vi "SERIAL_StartStreamCommand.vi"(11 "navX Ref":T1={"SerialPortRef"={"DevStatus"={"status"=FALSE, "code"=0, "source"=""}, "Serial Port Name"=""}, "Board Information"={"WhoAmI (50 | 0x32)"=0, "Board Revision"=0, "Firmware Major Version"=0, "Firmware Minor Version"=0, "NAVX_BOARD_CAPABILITY"={"OMNIMOUNT"=FALSE, "YAW_RESET"=FALSE, "VEL_AND_DISP"=FALSE}, "NAVX_BOARD_YAW_AXIS"={"BOARD_YAW_AXIS_UP"=FALSE, "BOARD_YAW_AXIS"=0}}, "Status"={"Update Rate Hz"=0, "Accelerometer Full-Scale Range"=0, "Gyro Full-Scale Range"=0, "NAVX_OP_STATUS"=0, "NAVX_CAL_STATUS"=0, "NAVX_SELFTEST_STATUS"=0, "NAVX_SENSOR_STATUS"={"MOVING"=FALSE, "YAW_STABLE"=FALSE, "MAG_DISTURBANCE"=FALSE, "ALTITUDE_VALID"=FALSE, "SEALEVEL_PRESS_SET"=FALSE, "FUSED_HEADING_VALID"=FALSE}}, "Offsets"={"Yaw"=0.0, "Quat W"=0.0, "Quat X"=0.0, "Quat Y"=0.0, "Quat Z"=0.0}, "Update Rate (4Hz-60Hz)"=50, "Nav6Mode (YPR)"=enum."Raw", "refnum name"="", "error"={"status"=FALSE, "code"=0, "source"=""}, "Loop VI Refnum"=refnum} {"Status"."NAVX_OP_STATUS" items=["INITIALIZING", "SELFTEST_IN_PROGRESS", "ERROR", "IMU_AUTOCAL_IN_PROGRESS", "NORMAL"]; "Status"."NAVX_CAL_STATUS" items=["IMU_CAL_STATE_MASK"=3, "IMU_CAL_INPROGRESS"=0, "IMU_CAL_ACCUMULATE"=1, "IMU_CAL_COMPLETE"=2, "MAG_CAL_COMPLETE"=4, "BARO_CAL_COMPLETE"=8]}) -> (3 "navX Ref":T1={"SerialPortRef"={"DevStatus"={"status"=FALSE, "code"=0, "source"=""}, "Serial Port Name"=""}, "Board Information"={"WhoAmI (50 | 0x32)"=0, "Board Revision"=0, "Firmware Major Version"=0, "Firmware Minor Version"=0, "NAVX_BOARD_CAPABILITY"={"OMNIMOUNT"=FALSE, "YAW_RESET"=FALSE, "VEL_AND_DISP"=FALSE}, "NAVX_BOARD_YAW_AXIS"={"BOARD_YAW_AXIS_UP"=FALSE, "BOARD_YAW_AXIS"=0}}, "Status"={"Update Rate Hz"=0, "Accelerometer Full-Scale Range"=0, "Gyro Full-Scale Range"=0, "NAVX_OP_STATUS"=0, "NAVX_CAL_STATUS"=0, "NAVX_SELFTEST_STATUS"=0, "NAVX_SENSOR_STATUS"={"MOVING"=FALSE, "YAW_STABLE"=FALSE, "MAG_DISTURBANCE"=FALSE, "ALTITUDE_VALID"=FALSE, "SEALEVEL_PRESS_SET"=FALSE, "FUSED_HEADING_VALID"=FALSE}}, "Offsets"={"Yaw"=0.0, "Quat W"=0.0, "Quat X"=0.0, "Quat Y"=0.0, "Quat Z"=0.0}, "Update Rate (4Hz-60Hz)"=50, "Nav6Mode (YPR)"=enum."Raw", "refnum name"="", "error"={"status"=FALSE, "code"=0, "source"=""}, "Loop VI Refnum"=refnum} {"Status"."NAVX_OP_STATUS" items=["INITIALIZING", "SELFTEST_IN_PROGRESS", "ERROR", "IMU_AUTOCAL_IN_PROGRESS", "NORMAL"]; "Status"."NAVX_CAL_STATUS" items=["IMU_CAL_STATE_MASK"=3, "IMU_CAL_INPROGRESS"=0, "IMU_CAL_ACCUMULATE"=1, "IMU_CAL_COMPLETE"=2, "MAG_CAL_COMPLETE"=4, "BARO_CAL_COMPLETE"=8]})   [LabVIEW 2014]
uses:
  navX Serial DevRef.ctl
  <vilib>/Rock Robotics/WPI/SerialPort/WPI_SerialPortRef.ctl
  COMMON/TypeDefs/Data TypeDefs/navX Board Information.ctl
  COMMON/TypeDefs/Value TypeDefs/navX NAVX_BOARD_CAPABILITY.ctl
  COMMON/TypeDefs/Value TypeDefs/navX NAVX_BOARD_YAW_AXIS.ctl
  COMMON/TypeDefs/Data TypeDefs/navX Status Data.ctl
  COMMON/TypeDefs/Value TypeDefs/navX NAVX_OP_STATUS.ctl
  COMMON/TypeDefs/Value TypeDefs/navX NAVX_CAL_STATUS.ctl
  COMMON/TypeDefs/Value TypeDefs/navX NAVX_SENSOR_STATUS.ctl
  COMMON/TypeDefs/Value TypeDefs/navX Serial Mode.ctl
  navX-MXP IMU.lvlib
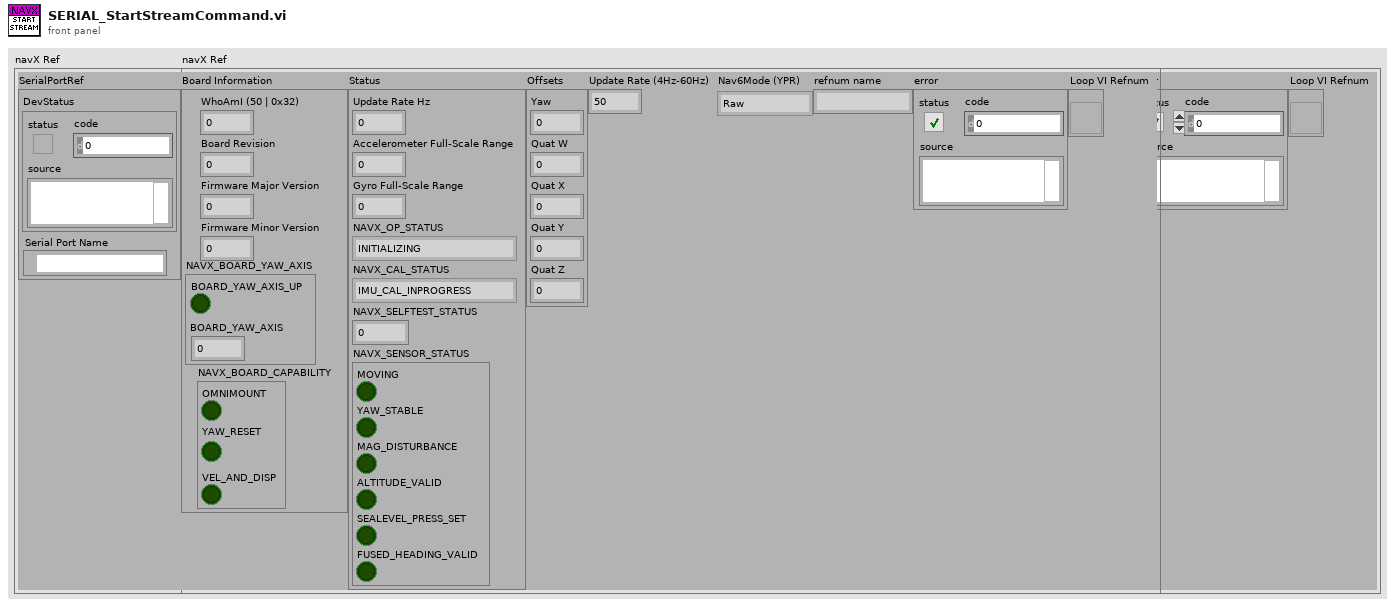
[diagram p1: front panel]
types:
  T1 = typedef "navX Serial DevRef.ctl" = cluster{"SerialPortRef":T2, "Board Information":T3, "Status":T6, "Offsets":cluster{"Yaw":dbl, "Quat W":dbl, "Quat X":dbl, "Quat Y":dbl, "Quat Z":dbl}, "Update Rate (4Hz-60Hz)":u8, "Nav6Mode (YPR)":T10, "refnum name":string, "error":errorcluster, "Loop VI Refnum":refnum<vi>}
  T2 = typedef "WPI_SerialPortRef.ctl" = cluster{"DevStatus":errorcluster, "Serial Port Name":refnum<visa-resource-name>}
  T3 = typedef "navX-MXP IMU.lvlib/navX Board Information.ctl" = cluster{"WhoAmI (50 | 0x32)":u8, "Board Revision":u8, "Firmware Major Version":u8, "Firmware Minor Version":u8, "NAVX_BOARD_CAPABILITY":T4, "NAVX_BOARD_YAW_AXIS":T5}
  T4 = typedef "navX-MXP IMU.lvlib/navX NAVX_BOARD_CAPABILITY.ctl" = cluster{"OMNIMOUNT":bool, "YAW_RESET":bool, "VEL_AND_DISP":bool}
  T5 = typedef "navX-MXP IMU.lvlib/navX NAVX_BOARD_YAW_AXIS.ctl" = cluster{"BOARD_YAW_AXIS_UP":bool, "BOARD_YAW_AXIS":u8}
  T6 = typedef "navX-MXP IMU.lvlib/navX Status Data.ctl" = cluster{"Update Rate Hz":u8, "Accelerometer Full-Scale Range":u8, "Gyro Full-Scale Range":u16, "NAVX_OP_STATUS":T7, "NAVX_CAL_STATUS":T8, "NAVX_SELFTEST_STATUS":u8, "NAVX_SENSOR_STATUS":T9}
  T7 = typedef "navX-MXP IMU.lvlib/navX NAVX_OP_STATUS.ctl" = u8
  T8 = typedef "navX-MXP IMU.lvlib/navX NAVX_CAL_STATUS.ctl" = u8
  T9 = typedef "navX-MXP IMU.lvlib/navX NAVX_SENSOR_STATUS.ctl" = cluster{"MOVING":bool, "YAW_STABLE":bool, "MAG_DISTURBANCE":bool, "ALTITUDE_VALID":bool, "SEALEVEL_PRESS_SET":bool, "FUSED_HEADING_VALID":bool}
  T10 = typedef "navX-MXP IMU.lvlib/navX Serial Mode.ctl" = enum16{"Raw", "Processed"}
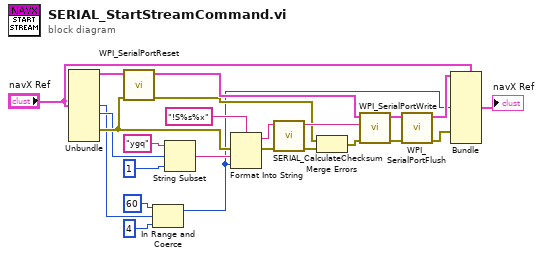
[diagram p0: block diagram]
diagram:
  n1 = Unbundle("navX Ref") -> ("SerialPortRef"=w24:T2, "Update Rate (4Hz-60Hz)"=w3:u8, "Nav6Mode (YPR)"=w4:T10, "error"=w5:errorcluster)  [unwired: 5 out]
  n2 = call <vilib>:"WPI_SerialPortReset.vi"("error in (no error)"=w5, "SerialPortRef"=w24) -> ("error out"=w10:errorcluster, "SerialPortRef"=w23:T2)  [unwired: 8 in]
  n3 = In Range and Coerce(upper limit=60, x=w3, lower limit=4) -> (coerced(x)=w2:i32)  [unwired: 1 out]
  n4 = String Subset(string="ygq", offset (0)=w4, length (rest)=1 ("length (rest)")) -> (substring=w13:string)
  n5 = Format Into String(format string="!S%s%x", error in=w5, w13, w2) -> (resulting string=w12:string, error out=w8:errorcluster)  [unwired: 1 in]
  n6 = call "SERIAL_CalculateChecksum.vi"("error in"=w8, "Content"=w12) -> ("error out"=w7:errorcluster, "Teminated Content"=w11:string)  [unwired: 4 in]
  n7 = Merge Errors(w10, w7) -> (w9:errorcluster)
  n8 = call <vilib>:"WPI_SerialPortWrite.vi"("error in (no error)"=w9, "Buffer"=w11, "SerialPortRef"=w23) -> ("error out"=w22:errorcluster, "SerialPortRef"=w21:T2)  [unwired: 6 in, 1 out]
  n9 = call <vilib>:"WPI_SerialPortFlush.vi"("error in (no error)"=w22, "SerialPortRef"=w21) -> ("error out"=w1:errorcluster, "SerialPortRef"=w17:T2)  [unwired: 8 in]
  n10 = Bundle(cluster="navX Ref", "SerialPortRef"=w17, "Update Rate (4Hz-60Hz)"=w2, "error"=w1) -> (→"navX Ref":T1)  [unwired: 6 in]
